vi "Calls VI In An LLB.vi"() -> (0 "error out":errorcluster, 2 "binary array":u32[](array[numeric]), 3 "Digital Waveform Graph":digitalwaveform(graph))   [LabVIEW 2013]
uses:
  <vilib>/Waveform/DWDTOps.llb/Digital Pattern Generator (Marching Values).vi
  <vilib>/Waveform/DWDTOps.llb/DWDT Digital to Binary U32.vi
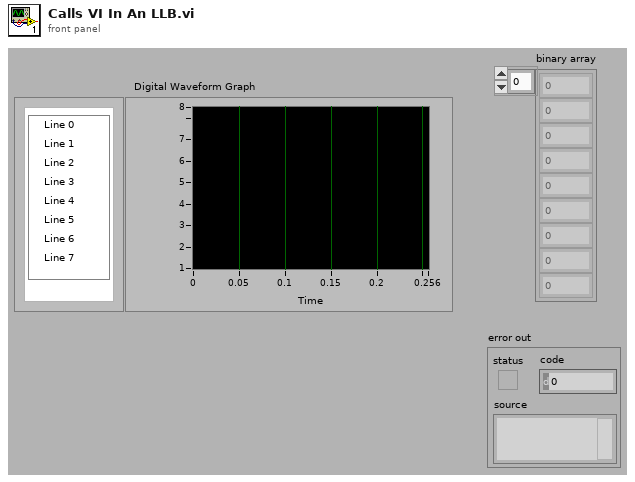
[diagram p1: front panel]
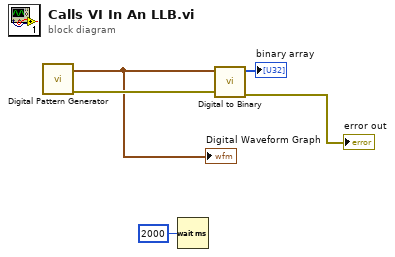
[diagram p0: block diagram]
diagram:
  n1 = call-poly <vilib>:"Digital Pattern Generator.vi"() -> ("error out"=w5:errorcluster, "digital waveform"=w2:digitalwaveform)  [unwired: 6 in, 4 out]
  "Digital Waveform Graph" <- w2
  n2 = Wait (ms)(milliseconds to wait=u32 2000) -> ()  [unwired: 1 out]
  n3 = call-poly <vilib>:"Digital to Binary.vi"("error in (no error)"=w5, "digital waveform"=w2) -> ("error out"=→"error out":errorcluster, "binary array"=→"binary array":u32[])  [unwired: 8 out]
